vi "Fpga-Exercisor-Top.vi"() -> ()   [LabVIEW 2017]
uses:
  <vilib>/Platform/TimedLoop/XDataNode/timing_clust.ctl
  <vilib>/Platform/TimedLoop/XDataNode/nitl_modes.ctl
  <vilib>/Platform/TimedLoop/XDataNode/wakeup.ctl
  <vilib>/rvi/Emulation/niFpgaSctlEmulationGetInTimedLoop.vi
  <vilib>/rvi/Emulation/niFpgaEmulationReportErrorSimple.vi
  <vilib>/rvi/Emulation/niFpgaGetClockAttributes.vi
  <vilib>/rvi/Emulation/niFpgaCriticalErrorInLSC.vi
  <vilib>/rvi/interface/RandomDataEmulation/niFpgaRandomDataHandleErrors.vi
  <vilib>/rvi/eio/common/nirviEmuTemplateMethod_errors.vi
  <vilib>/Platform/TimedLoop/XDataNode/XDataNode.xnode
  <vilib>/rvi/DataTransferAndStorage/Container/XNode/niFpgaContainer.xnode
  <vilib>/rvi/interface/RandomDataEmulation/nirviRandomDataFpgaReadWriteTemplate.vi
  <vilib>/eio/EIONode/EIONode.xnode
  <vilib>/Platform/TimedLoop/XDataNode/XDNodeRunTimeDep.lvlib
panel:
  out "AXI_STR_RXD_tready 3":bool
  out "tvalid 3":bool
  out "tdata 3":u32
  out "tlast 3":bool
  out "AXI_STR_RXD_tready_Count 3":u16
  out "tvalid_Count 3":u16
  out "tlast_Count 3":u16
  out "tdata_LastNonZero 3":u32
  out "AXI_STR_RXD_tready 2":bool
  out "tvalid 2":bool
  out "tdata 2":u32
  out "tlast 2":bool
  out "AXI_STR_RXD_tready_Count 2":u16
  out "tvalid_Count 2":u16
  out "tlast_Count 2":u16
  out "tdata_LastNonZero 2":u32
  in  "Interrupt #1":bool
  in  "Interrupt #0":bool
  out "GPIO #2 out":u32
  in  "GPIO #2 in":u32
  out "GPIO #1 out":u32
  in  "GPIO #1 in":u32
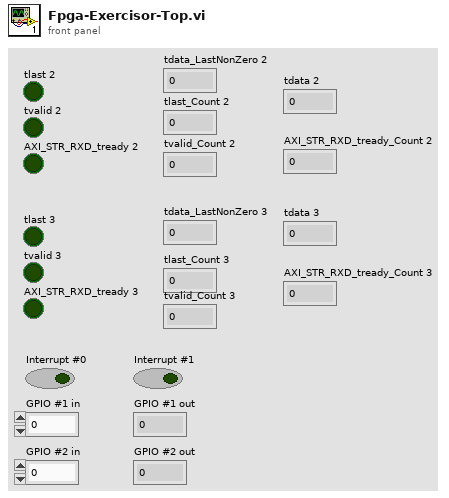
[diagram p1: front panel]
types:
  T1 = typedef "XDNodeRunTimeDep.lvlib/timing_clust.ctl" = cluster{"Expected End [f-1]":u64, "Actual End [f-1]":u64, "Finished Late? [f-1]":bool, "Expected End [i-1]":u64, "Actual End [i-1]":u64, "Finished Late? [i-1]":bool, "Expected Start [i]":u64, "Actual Start [i]":u64, "Expected Start [f]":u64, "Actual Start [f]":u64, "Source Name":string, "Structure Name":string, "Period":i64, "Deadline":i64, "Offset":i64, "Start":i64, "Priority":i32, "Timeout":i32, "Mode":T2, "Wakeup Reason":T3, "Error":errorcluster, "Source Type":string, "Secondary Source Type":string, "Global End Time":u64, "Global Start Time":u64, "Frame Duration":u64, "Iteration Duration":u64, "Assigned CPU":i32, "I/O Scan Engine Mode":u32}
  T2 = typedef "XDNodeRunTimeDep.lvlib/nitl_modes.ctl" = enum32{"No Change", "Process missed periods, maintain original phase", "Discard missed periods, maintain original phase", "Process missed periods, ignore original phase", "Discard missed periods, ignore original phase"}
  T3 = typedef "XDNodeRunTimeDep.lvlib/wakeup.ctl" = enum32{"Normal", "Aborted", "Asynchronous wakeup", "Timing source error", "Timed loop error", "Timeout"}
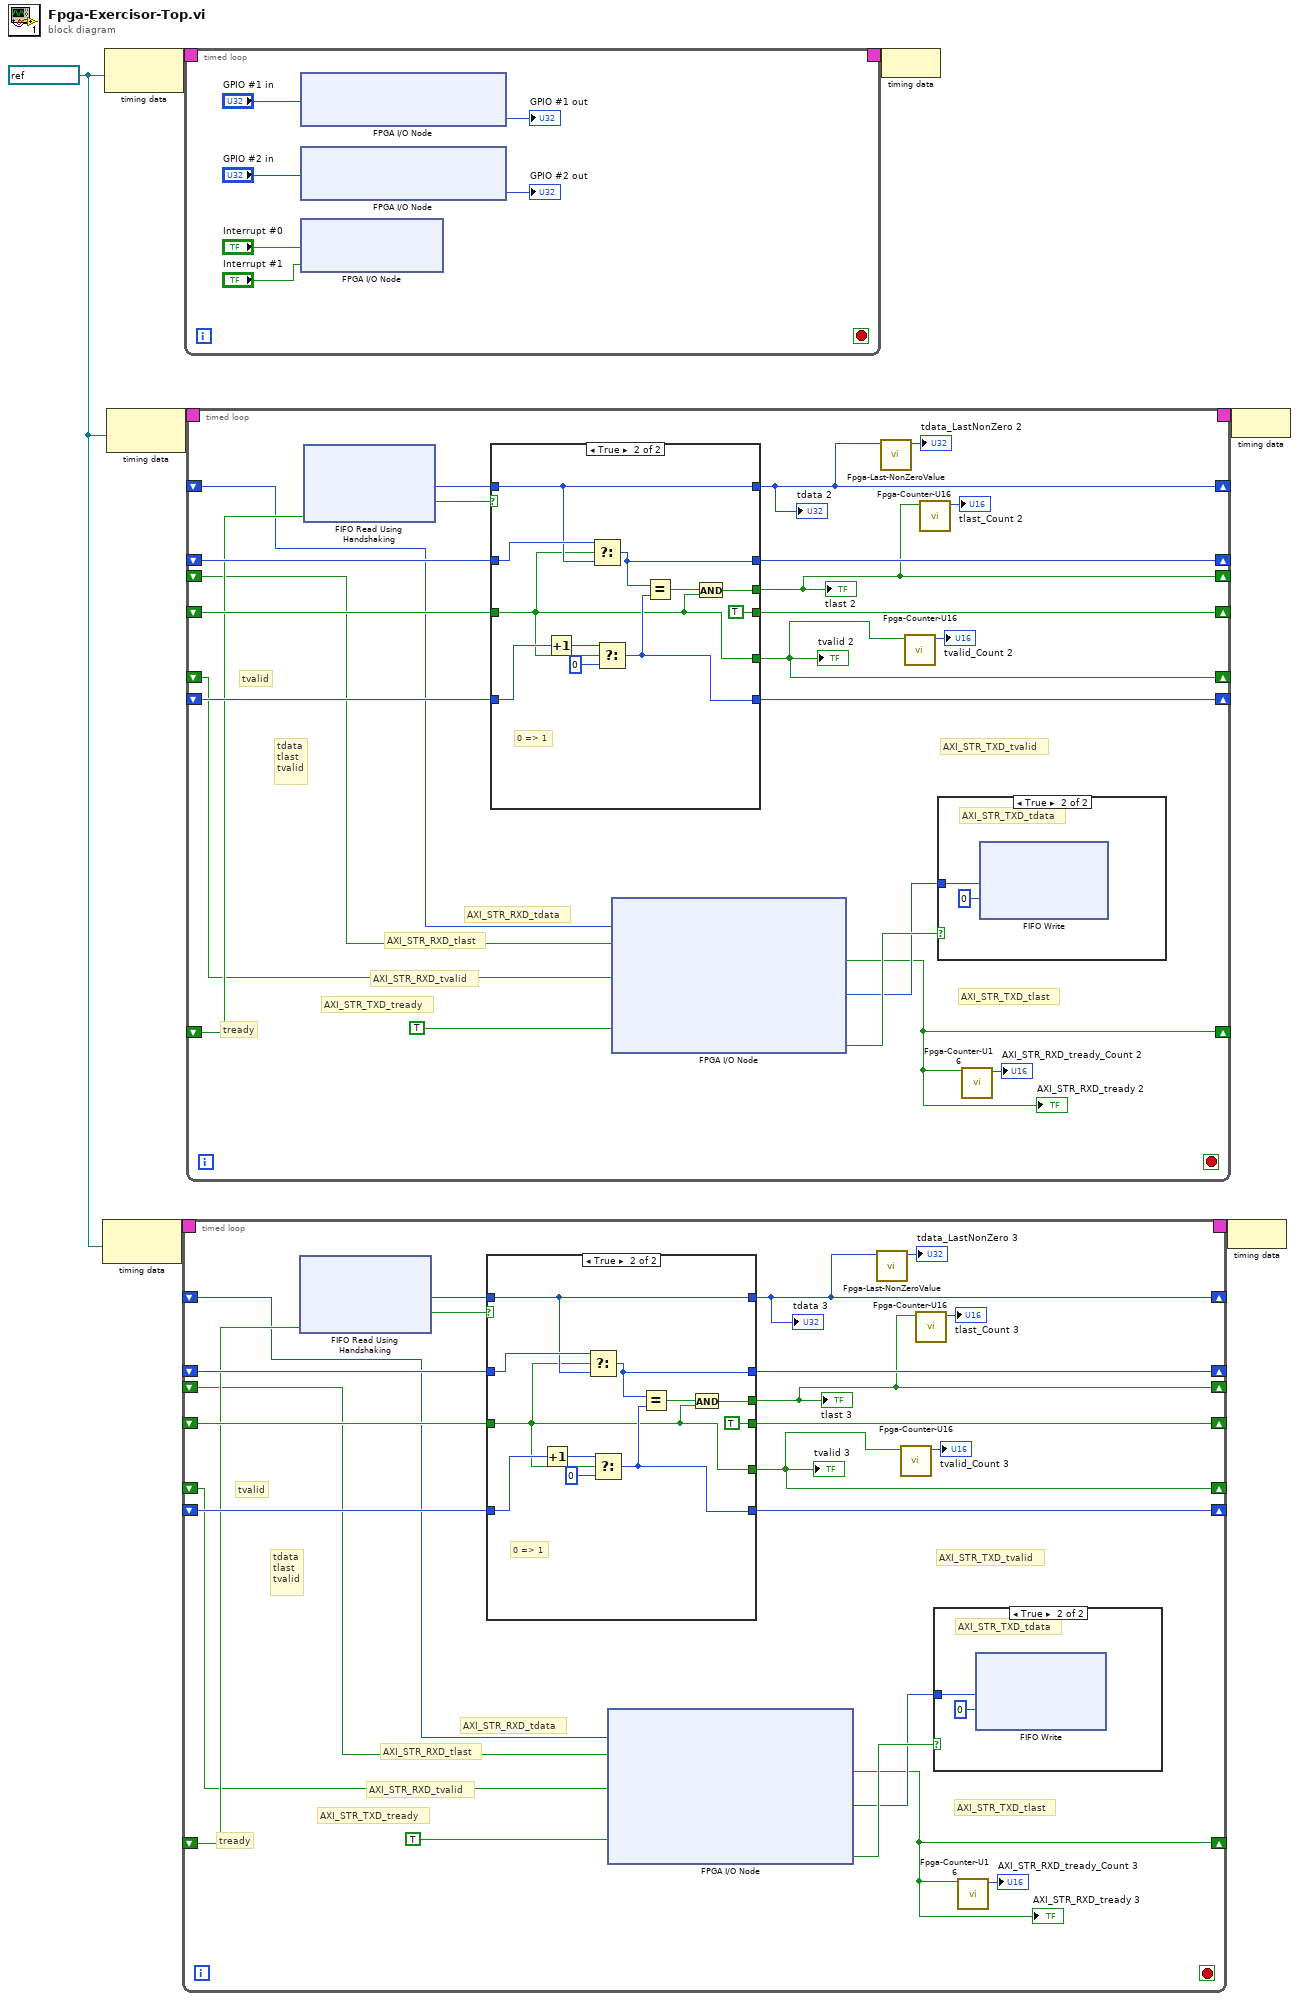
[diagram p0: block diagram]
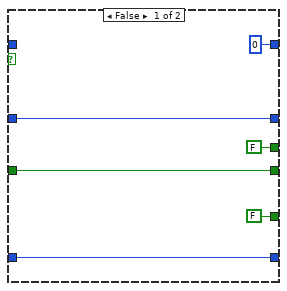
[diagram p3: hidden frame]
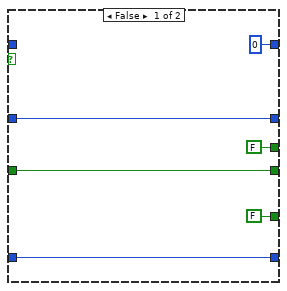
[diagram p5: hidden frame]
diagram:
  w1 = refnum<k21> "100MHz" ("Source Name")
  n1 = node-c288(w1) -> (w3:T1)
  n2 = node-c288(w1) -> (w7:T1)
  n3 = node-c288(w1) -> (w5:T1)
  n4 = timed-loop {
    timing: w3 -> [_]
    timing-out: [_] -> w2
    shift-right: [w28] -> _
    shift-left: _ -> [w29]
    shift-right: [w25] -> _
    shift-left: _ -> [w27]
    shift-right: [w23] -> _
    shift-left: _ -> [w24]
    shift-right: [w20] -> _
    shift-left: _ -> [w12]
    shift-right: [w8] -> _
    shift-left: _ -> [w22]
    shift-right: [w16] -> _
    shift-left: _ -> [w14]
    shift-right: [w18] -> _
    shift-left: _ -> [w13]
    stop <- _ stop-if-true
    # "AXI_STR_TXD_tlast"
    # "AXI_STR_TXD_tvalid"
    # "AXI_STR_TXD_tready"
    # "AXI_STR_RXD_tvalid"
    # "AXI_STR_RXD_tlast"
    # "AXI_STR_RXD_tdata"
    # "tvalid"
    # "tready"
    # "tdata\ntlast\ntvalid"
    n5 = xnode ("FIFO Read Using Handshaking")("Ready for Output"=w22) -> ("Element"=w26:u32, "Output Valid"=w30:bool)  [unwired: 1 in, 1 out]
    n6 = case shown="True" w30 {
      tunnel: w29 -> [w37 w39]
      tunnel: [w37 TRUE ("Size\nRead?")] -> w28
      tunnel: w27 -> [w38 w49]
      tunnel: w26 -> [_ w44]
      tunnel: [w38 w43] -> w25
      tunnel: w24 -> [w36 w48]
      tunnel: [w36 w42] -> w23
      tunnel: [FALSE ("Size\nRead?") w39] -> w20
      tunnel: [u32 0 ("Element") w44] -> w16
      tunnel: [FALSE w40] -> w18
      frame False {
      }
      frame True {
        # "0 => 1"
        n7 = Increment(x=w48) -> (x+1=w46:u32)
        n8 = Select(t=w49, s=w39, f=w44) -> (s? t:f=w43:u32)
        n9 = Select(t=w46, s=w39, f=u32 0) -> (s? t:f=w42:u32)
        n10 = Equal?(x=w43, y=w42) -> (x = y?=w41:bool)
        n11 = And(x=w41, y=w39) -> (x .and. y?=w40:bool)
      }
    }
    "tvalid 3" <- w20
    "tdata 3" <- w16
    "tlast 3" <- w18
    n12 = xnode "FPGA I/O Node"("d_microblaze_i\\AXI_STR_RXD_1_tdata"=w14, "d_microblaze_i\\AXI_STR_RXD_1_tlast"=w13, "d_microblaze_i\\AXI_STR_RXD_1_tvalid"=w12, "d_microblaze_i\\AXI_STR_TXD_1_tready"=TRUE ("d_microblaze\\AXI_STR_TXD_tready")) -> ("d_microblaze_i\\AXI_STR_RXD_1_tready"=w8:bool, "d_microblaze_i\\AXI_STR_TXD_1_tdata"=w9:u32, "d_microblaze_i\\AXI_STR_TXD_1_tvalid"=w10:bool)  [unwired: 8 in, 9 out]
    "AXI_STR_RXD_tready 3" <- w8
    n13 = call "Fpga-Last-NonZeroValue.vi"("d_mcs_i\\IO_BUS_write_data in"=w16) -> ("d_mcs_i\\IO_BUS_write_data out"=→"tdata_LastNonZero 3":u32)  [unwired: 10 in]
    n14 = call "Fpga-Counter-U16.vi"("d_mcs_i\\IO_BUS_read_strobe"=w20) -> ("Numeric"=→"tvalid_Count 3":u16)  [unwired: 10 in]
    n15 = call "Fpga-Counter-U16.vi"("d_mcs_i\\IO_BUS_read_strobe"=w18) -> ("Numeric"=→"tlast_Count 3":u16)  [unwired: 10 in]
    n16 = case shown="True" w10 {
      tunnel: w9 -> [_ w32]
      frame False {
      }
      frame True {
        # "AXI_STR_TXD_tdata"
        n17 = xnode ("FIFO Write")("Element"=w32, "Timeout"=0) -> ()  [unwired: 1 in, 2 out]
      }
    }
    n18 = call "Fpga-Counter-U16.vi"("d_mcs_i\\IO_BUS_read_strobe"=w8) -> ("Numeric"=→"AXI_STR_RXD_tready_Count 3":u16)  [unwired: 10 in]
  }
  n19 = timed-loop {
    timing: w7 -> [_]
    timing-out: [_] -> w6
    stop <- _ stop-if-true
    n20 = xnode "FPGA I/O Node"("d_microblaze_i\\gpio_rtl_tri_i"="GPIO #1 in") -> ("d_microblaze_i\\gpio_rtl_0_tri_o"=→"GPIO #1 out":u32)  [unwired: 2 in, 2 out]
    n21 = xnode "FPGA I/O Node"("d_microblaze_i\\gpio_rtl_1_tri_i"="GPIO #2 in") -> ("d_microblaze_i\\gpio_rtl_2_tri_o"=→"GPIO #2 out":u32)  [unwired: 2 in, 2 out]
    n22 = xnode "FPGA I/O Node"("d_microblaze_i\\In0"="Interrupt #0", "d_microblaze_i\\In1"="Interrupt #1") -> ()  [unwired: 2 in, 2 out]
  }
  n23 = timed-loop {
    timing: w5 -> [_]
    timing-out: [_] -> w4
    shift-right: [w80] -> _
    shift-left: _ -> [w81]
    shift-right: [w77] -> _
    shift-left: _ -> [w79]
    shift-right: [w75] -> _
    shift-left: _ -> [w76]
    shift-right: [w72] -> _
    shift-left: _ -> [w64]
    shift-right: [w60] -> _
    shift-left: _ -> [w74]
    shift-right: [w68] -> _
    shift-left: _ -> [w66]
    shift-right: [w70] -> _
    shift-left: _ -> [w65]
    stop <- _ stop-if-true
    # "AXI_STR_TXD_tlast"
    # "AXI_STR_TXD_tvalid"
    # "AXI_STR_TXD_tready"
    # "AXI_STR_RXD_tvalid"
    # "AXI_STR_RXD_tlast"
    # "AXI_STR_RXD_tdata"
    # "tvalid"
    # "tready"
    # "tdata\ntlast\ntvalid"
    n24 = xnode ("FIFO Read Using Handshaking")("Ready for Output"=w74) -> ("Element"=w78:u32, "Output Valid"=w82:bool)  [unwired: 1 in, 1 out]
    n25 = case shown="True" w82 {
      tunnel: w81 -> [w89 w91]
      tunnel: [w89 TRUE ("Size\nRead?")] -> w80
      tunnel: w79 -> [w90 w101]
      tunnel: w78 -> [_ w96]
      tunnel: [w90 w95] -> w77
      tunnel: w76 -> [w88 w100]
      tunnel: [w88 w94] -> w75
      tunnel: [FALSE ("Size\nRead?") w91] -> w72
      tunnel: [u32 0 ("Element") w96] -> w68
      tunnel: [FALSE w92] -> w70
      frame False {
      }
      frame True {
        # "0 => 1"
        n26 = Increment(x=w100) -> (x+1=w98:u32)
        n27 = Select(t=w101, s=w91, f=w96) -> (s? t:f=w95:u32)
        n28 = Select(t=w98, s=w91, f=u32 0) -> (s? t:f=w94:u32)
        n29 = Equal?(x=w95, y=w94) -> (x = y?=w93:bool)
        n30 = And(x=w93, y=w91) -> (x .and. y?=w92:bool)
      }
    }
    "tvalid 2" <- w72
    "tdata 2" <- w68
    "tlast 2" <- w70
    n31 = xnode "FPGA I/O Node"("d_microblaze_i\\AXI_STR_RXD_tdata"=w66, "d_microblaze_i\\AXI_STR_RXD_tlast"=w65, "d_microblaze_i\\AXI_STR_RXD_tvalid"=w64, "d_microblaze_i\\AXI_STR_TXD_tready"=TRUE ("d_microblaze\\AXI_STR_TXD_tready")) -> ("d_microblaze_i\\AXI_STR_RXD_tready"=w60:bool, "d_microblaze_i\\AXI_STR_TXD_tdata"=w61:u32, "d_microblaze_i\\AXI_STR_TXD_tvalid"=w62:bool)  [unwired: 8 in, 9 out]
    "AXI_STR_RXD_tready 2" <- w60
    n32 = call "Fpga-Last-NonZeroValue.vi"("d_mcs_i\\IO_BUS_write_data in"=w68) -> ("d_mcs_i\\IO_BUS_write_data out"=→"tdata_LastNonZero 2":u32)  [unwired: 10 in]
    n33 = call "Fpga-Counter-U16.vi"("d_mcs_i\\IO_BUS_read_strobe"=w72) -> ("Numeric"=→"tvalid_Count 2":u16)  [unwired: 10 in]
    n34 = call "Fpga-Counter-U16.vi"("d_mcs_i\\IO_BUS_read_strobe"=w70) -> ("Numeric"=→"tlast_Count 2":u16)  [unwired: 10 in]
    n35 = case shown="True" w62 {
      tunnel: w61 -> [_ w84]
      frame False {
      }
      frame True {
        # "AXI_STR_TXD_tdata"
        n36 = xnode ("FIFO Write")("Element"=w84, "Timeout"=0) -> ()  [unwired: 1 in, 2 out]
      }
    }
    n37 = call "Fpga-Counter-U16.vi"("d_mcs_i\\IO_BUS_read_strobe"=w60) -> ("Numeric"=→"AXI_STR_RXD_tready_Count 2":u16)  [unwired: 10 in]
  }
  n38 = node-c288(w6) -> ()
  n39 = node-c288(w2) -> ()
  n40 = node-c288(w4) -> ()
